vi "FP_QTMTelegram_Write.vi"(3 "error in (no error)":errorcluster, 4 "timeout ms (25000)":i32, 5 "String to send":string, 6 "connection ID":refnum<k5>) -> (0 "error out":errorcluster, 1 "bytes written":i32, 2 "connection ID out":refnum<k5>)   [LabVIEW 2010]
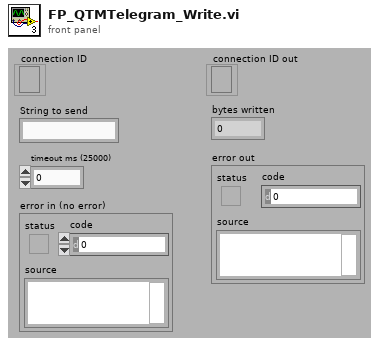
[diagram p1: front panel]
types:
  T1 = enum16{"big-endian, network order", "native, host order", "little-endian"}
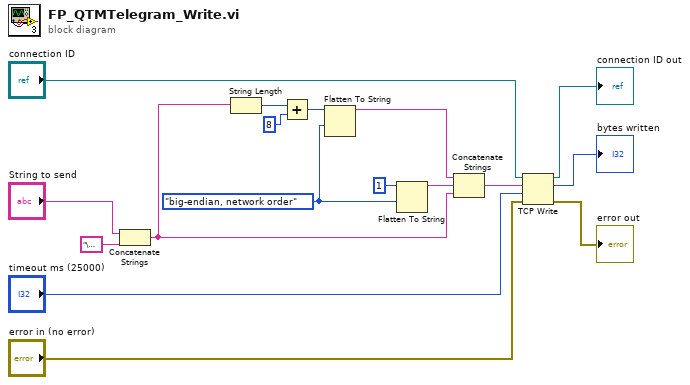
[diagram p0: block diagram]
diagram:
  w13 = T1."big-endian, network order" ("byte order (0:big-endian, network order)")
  n1 = Concatenate Strings("String to send", "\u0000") -> (w9:string)
  n2 = String Length(string=w9) -> (length=w12:i32)
  n3 = Add(x=w12, y=8) -> (x+y=w15:i32)
  n4 = Flatten To String(anything=w15, byte order (0:big-endian, network order)=w13) -> (data string=w10:string)  [unwired: 1 in, 3 out]
  n5 = Flatten To String(anything=1, byte order (0:big-endian, network order)=w13) -> (data string=w11:string)  [unwired: 1 in, 3 out]
  n6 = Concatenate Strings(w10, w11, w9) -> (w8:string)
  n7 = TCP Write(connection ID="connection ID", data in=w8, error in (no error)="error in (no error)", 9:"timeout ms (25000)") -> (connection ID out=→"connection ID out":refnum<k5>, bytes written=→"bytes written":i32, error out=→"error out":errorcluster)
